vi "Array, Write Diagonal, DBL.vi"(1 "diagonal (1)":dbl=1.0 format="%.1f", 2 "col (0)":i32, 3 "row (0)":i32, 4 "array in":dbl[][](array[numeric]) format="%.1g") -> (0 "array out":dbl[][](array[numeric]) format="%.1g")   [LabVIEW 2010]
doc: "This function writes an element to the diagonal of an array. The start row and start column are optional.\nIf the start row or start column exceeds the dimensions of the input array, the array size will be increased to accomodate the new values."
uses:
  <vilib>/Analysis/Matrix/Numeric/Conversions/Array To Matrix - RA2.vi
  <vilib>/Analysis/Matrix/Numeric/Conversions/Matrix To Array - RM.vi
  <vilib>/Analysis/Matrix/NI_Matrix.lvlib
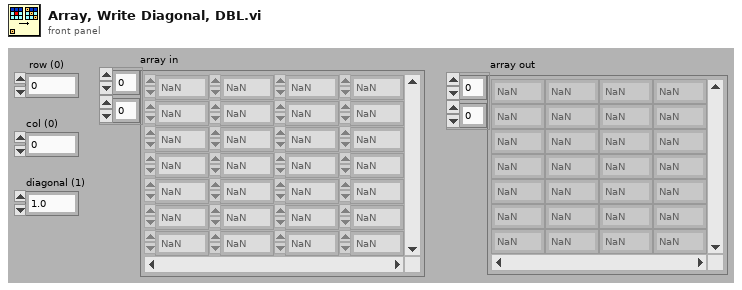
[diagram p1: front panel]
types:
  T1 = typedef "NI_Matrix.lvlib/RealMatrix.ctl" = dbl[][]
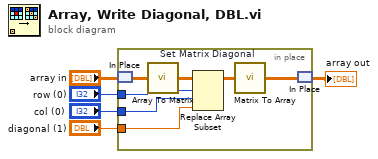
[diagram p0: block diagram]
diagram:
  n1 = in-place {
    in-place-border: "diagonal (1)" -> [w8]
    in-place-border: "col (0)" -> [w7]
    in-place-border: "row (0)" -> [w6]
    n2 = in-place-match #1("array in") -> (w10:dbl[][])
    n3 = call-poly <vilib>:"Array To Matrix.vi"("Real 2D Array"=w10) -> ("Real Matrix"=w11:T1)
    n4 = Replace Array Subset "Set Matrix Diagonal"(array=w11, new element=w8, index (row)=w6, index (col)=w7) -> (w12:T1)
    n5 = call-poly <vilib>:"Matrix To Array.vi"("Real Matrix"=w12) -> ("Real 2D Array"=w9:dbl[][])
    n6 = in-place-match #1(w9) -> (→"array out":dbl[][])
  }
